vi "SetMatlabTempParamData.vi"(8 "index in":dbl=-1.0, 10 "Matlab param data":T1[](array[typedef]), 11 "ExperimentID":string) -> (3 "index out":dbl)   [LabVIEW 2017]
uses:
  Types/MatlabDataBundle.ctl
  Types/MatlabDataType.ctl
  Types/MatlabDataContainerType.ctl
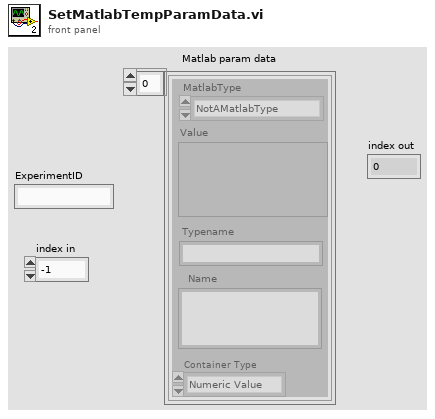
[diagram p1: front panel]
types:
  T1 = typedef "MatlabDataBundle.ctl" = cluster{"MatlabType":T2, "Value":variant, "Name":string, "Typename":string, "Container Type":T3}
  T2 = typedef "MatlabDataType.ctl" = enum16{"NotAMatlabType", "Real", "Complex", "String", "Boolean"}
  T3 = typedef "MatlabDataContainerType.ctl" = enum16{"Numeric Value", "Numeric Array", "Waveform"}
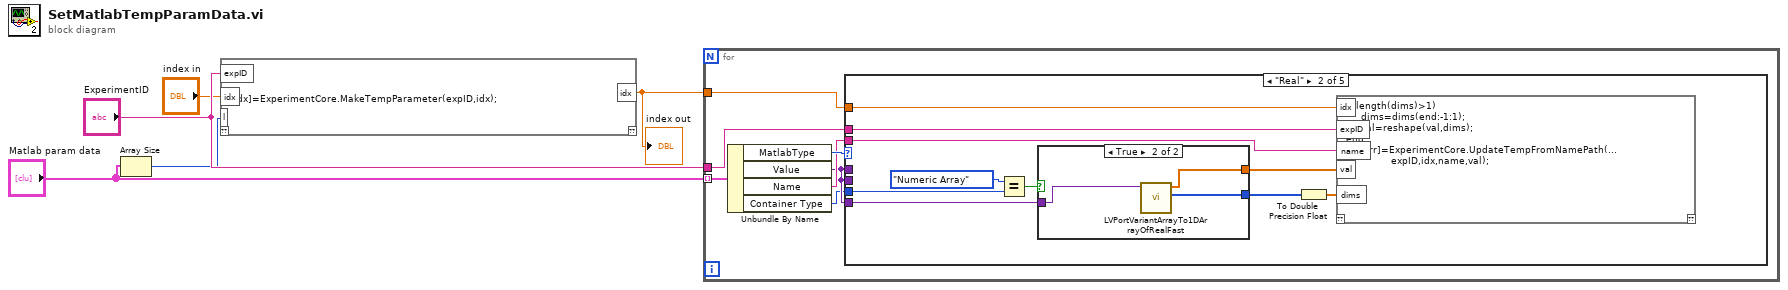
[diagram p0: block diagram]
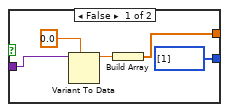
[diagram p3: hidden frame]
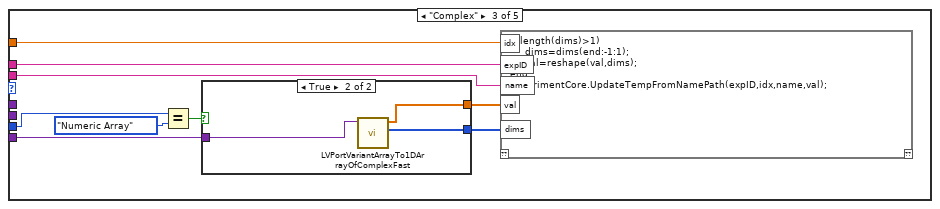
[diagram p4: hidden frame]
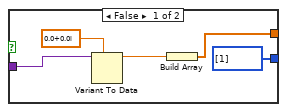
[diagram p5: hidden frame]
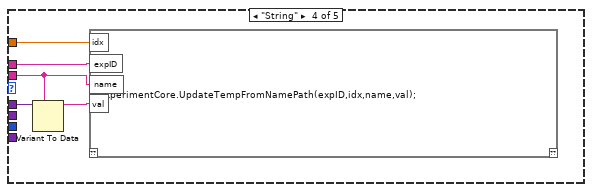
[diagram p6: hidden frame]
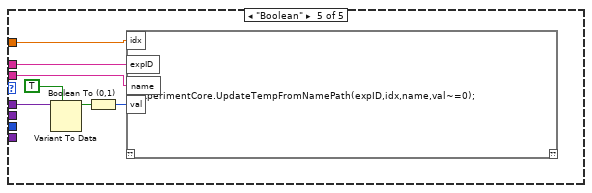
[diagram p7: hidden frame]
diagram:
  n1 = Array Size(array="Matlab param data") -> (size(s)=w1:i32)
  n2 = script code="[idx]=ExperimentCore.MakeTempParameter(expID,idx);"("expID"="ExperimentID", "idx"="index in", "l"=w1) -> ("idx"=w3:dbl)  [unwired: 1 in, 1 out]
  "index out" <- w3
  n3 = for {
    tunnel: "Matlab param data" -> [w11] mode=indexing
    tunnel: "ExperimentID" -> [w12]
    tunnel: w3 -> [w7]
    n4 = Unbundle By Name(w11) -> ("MatlabType"=w10:T2, "Value"=w8:variant, "Name"=w9:string, "Container Type"=w6:T3)
    n5 = case shown="\"Real\"" w10 {
      tunnel: w12 -> [_ w22 w35 w51 w56]
      tunnel: w8 -> [_ _ _ w52 w55]
      tunnel: w9 -> [_ w21 w33 w50 w54]
      tunnel: w8 -> [_ _ _ _ _]
      tunnel: w8 -> [_ w19 w38 _ _]
      tunnel: w7 -> [_ w16 w34 w48 w53]
      tunnel: w6 -> [_ w15 w32 _ _]
      frame "NotAMatlabType", Default {
      }
      frame "Real" {
        n6 = Equal?(x=MatlabDataContainerType."Numeric Array", y=w15) -> (x = y?=w13:bool)
        n7 = case shown="True" w13 {
          tunnel: [w25 w29] -> w20
          tunnel: w19 -> [w23 w30]
          tunnel: [u32[] [1] ("Size(s)") w28] -> w18
          frame False {
            n8 = Variant To Data(type=0.0, Variant=w23) -> (data=w26:dbl)  [unwired: 1 in, 1 out]
            n9 = Build Array(w26) -> (w25:dbl[])
          }
          frame True {
            n10 = call "LVPortVariantArrayTo1DArrayOfRealFast.vi"("Variant Real Array"=w30) -> ("Size(s)"=w28:u32[], "1D Array"=w29:dbl[])  [unwired: 8 in, 1 out]
          }
        }
        n11 = To Double Precision Float(number=w18) -> (double precision float=w17:dbl[])
        n12 = script code="if(length(dims)>1)\n     dims=dims(end:-1:1);\n     val=reshape(val,dims);\nend\n[strErr]=ExperimentCore.UpdateTempFromNamePath(...\n               expID,idx,name,val);"("expID"=w22, "name"=w21, "val"=w20, "dims"=w17, "idx"=w16) -> ()  [unwired: 1 in, 1 out]
      }
      frame "Complex" {
        n13 = Equal?(x=w32, y=MatlabDataContainerType."Numeric Array") -> (x = y?=w39:bool)
        n14 = case shown="True" w39 {
          tunnel: [w43 w46] -> w36
          tunnel: w38 -> [w41 w47]
          tunnel: [u32[] [1] ("Size(s)") w45] -> w37
          frame False {
            n15 = Variant To Data(type=cdb 0.0+0.0i, Variant=w41) -> (data=w44:cdb)  [unwired: 1 in, 1 out]
            n16 = Build Array(w44) -> (w43:cdb[])
          }
          frame True {
            n17 = call "LVPortVariantArrayTo1DArrayOfComplexFast.vi"("Variant Real Array"=w47) -> ("Size(s)"=w45:u32[], "1D Array"=w46:cdb[])  [unwired: 8 in, 1 out]
          }
        }
        n18 = script code="if(length(dims)>1)\n     dims=dims(end:-1:1);\n     val=reshape(val,dims);\nend\nExperimentCore.UpdateTempFromNamePath(expID,idx,name,val);"("expID"=w35, "name"=w33, "val"=w36, "dims"=w37, "idx"=w34) -> ()  [unwired: 1 in, 1 out]
      }
      frame "String" {
        n19 = Variant To Data(type=w50, Variant=w52) -> (data=w49:string)  [unwired: 1 in, 1 out]
        n20 = script code="ExperimentCore.UpdateTempFromNamePath(expID,idx,name,val);"("expID"=w51, "name"=w50, "val"=w49, "idx"=w48) -> ()  [unwired: 1 in, 1 out]
      }
      frame "Boolean" {
        n21 = Variant To Data(type=TRUE, Variant=w55) -> (data=w58:bool)  [unwired: 1 in, 1 out]
        n22 = Boolean To (0,1)(Boolean=w58) -> (0, 1=w57:i16)
        n23 = script code="ExperimentCore.UpdateTempFromNamePath(expID,idx,name,val~=0);"("expID"=w56, "name"=w54, "val"=w57, "idx"=w53) -> ()  [unwired: 1 in, 1 out]
      }
    }
  }
